vi "getSweepStatus.vi"(8 "error in (no error)":errorcluster, 10 "sweep status":T1=enum."sweeping", 11 "Generator in":refnum<class "Generator.lvclass">) -> (0 "error out":errorcluster, 3 "Generator out":refnum<class "Generator.lvclass">)   [LabVIEW 2019, in "Generator.lvclass"]
uses:
  Generator.lvclass
  typedefs/Generator.Sweep Status--enum.ctl
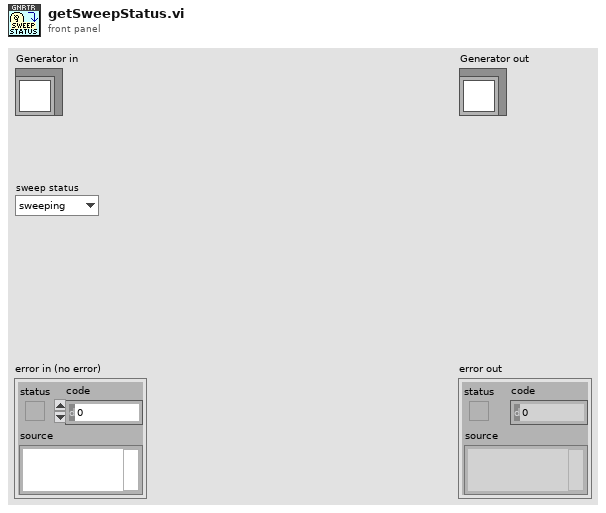
[diagram p1: front panel]
types:
  T1 = typedef "Generator.lvclass/Generator.Sweep Status--enum.ctl" = enum16{"idle", "initializing", "waiting", "sweeping", "stopping"}
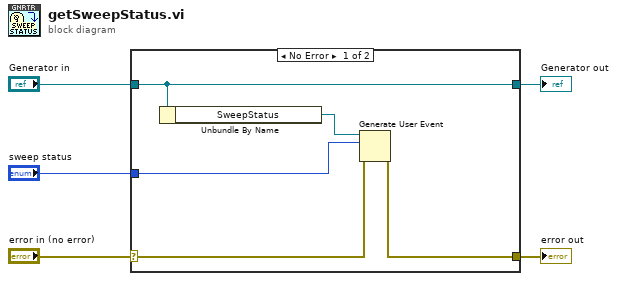
[diagram p0: block diagram]
diagram:
  n1 = case shown="No Error" "error in (no error)" {
    selector: "error in (no error)" -> [w9 w11]
    tunnel: [w8 w11] -> w4
    tunnel: [w7 w12] -> w2
    tunnel: "Generator in" -> [w7 w12]
    tunnel: "sweep status" -> [w10 _]
    frame No Error {
      n2 = Unbundle By Name(w7) -> ("SweepStatus"=w6:refnum<user-event>)
      n3 = Generate User Event(user event=w6, event data cluster=w10, error in=w9) -> (error out=w8:errorcluster)  [unwired: 1 in, 1 out]
    }
    frame Error {
    }
  }
  "error out" <- w4
  "Generator out" <- w2
